vi "CAN_parse_BMS_1.vi"(11 "CAN message data":u8[](array[numeric])) -> ()   [LabVIEW 2018]
uses:
  Type_Def/TypeDef_BMSDatas.ctl
  Type_Def/TypeDef_BMSStatuss.ctl
  <vilib>/CANopenLib/CANOPEN.llb/CANopen Fetch from Data [U16].vi
  <vilib>/CANopenLib/CANOPEN.llb/CANopen Fetch from Data [I8].vi
panel:
  out "output cluster":T1
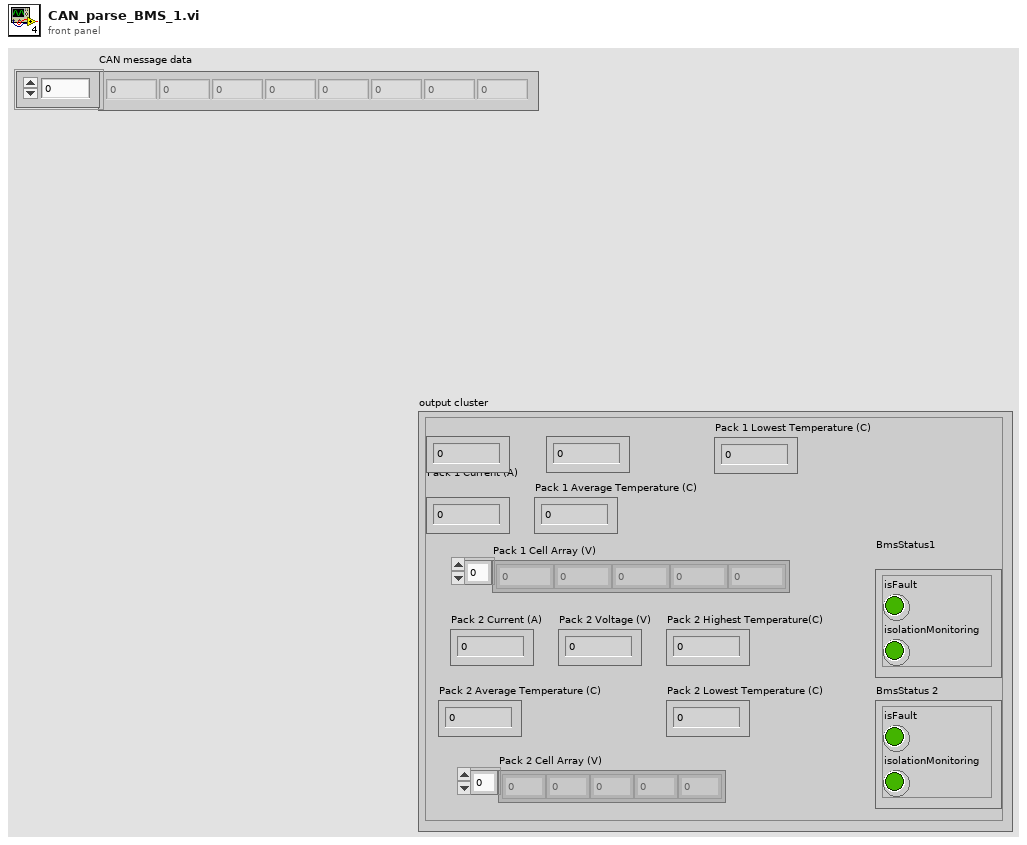
[diagram p1: front panel]
types:
  T1 = typedef "TypeDef_BMSDatas.ctl" = cluster{"Pack 1 Current (A)":dbl, "Pack 1 Voltage (V)":dbl, "Pack 1 Highest Temperature(C)":dbl, "BmsStatus1":T2, "Pack 2 Current (A)":dbl, "Pack 2 Voltage (V) ":dbl, "Pack 2 Highest Temperature(C) ":dbl, "BmsStatus 2":T2, "Pack 1 Cell Array (V)":dbl[], "Pack 2 Cell Array (V)":dbl[], "Pack 1 Lowest Temperature (C)":dbl, "Pack 1 Average Temperature (C)":dbl, "Pack 2 Average Temperature (C)":dbl, "Pack 2 Lowest Temperature (C)":dbl}
  T2 = typedef "TypeDef_BMSStatuss.ctl" = cluster{"isFault":bool, "isolationMonitoring":bool}
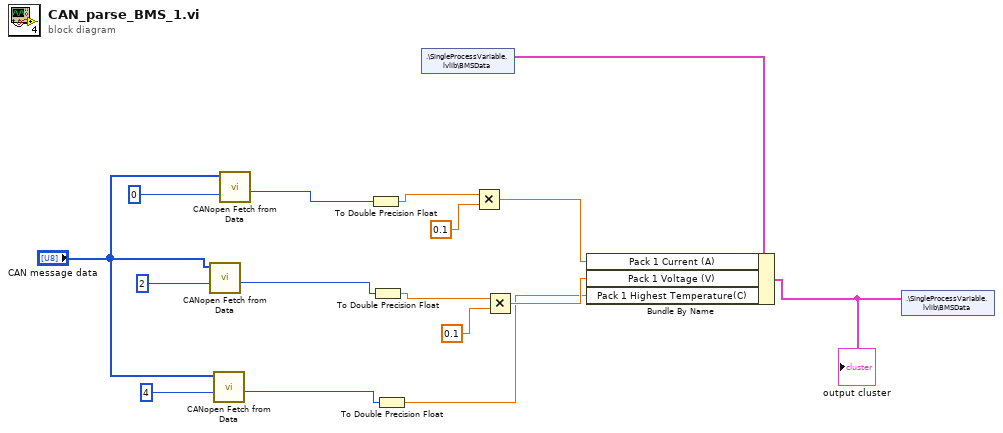
[diagram p0: block diagram]
diagram:
  n1 = call-poly <vilib>:"CANopen Fetch from Data.vi"("offset (0)"=2, "CANopen data in"="CAN message data") -> ("unsigned 16-bit integer"=w5:u16)  [unwired: 7 in, 2 out]
  n2 = call-poly <vilib>:"CANopen Fetch from Data.vi"("offset (0)"=4, "CANopen data in"="CAN message data") -> ("signed 8-bit integer"=w3:i8)  [unwired: 7 in, 2 out]
  n3 = call-poly <vilib>:"CANopen Fetch from Data.vi"("offset (0)"=0, "CANopen data in"="CAN message data") -> ("unsigned 16-bit integer"=w9:u16)  [unwired: 7 in, 2 out]
  n4 = To Double Precision Float(number=w9) -> (double precision float=w12:dbl)
  n5 = To Double Precision Float(number=w5) -> (double precision float=w6:dbl)
  n6 = To Double Precision Float(number=w3) -> (double precision float=w2:dbl)
  n7 = shared-variable ".\\SingleProcessVariable.lvlib\\BMSData"() -> (w14:T1)  [unwired: 1 in, 1 out]
  n8 = Multiply(x=w12, y=0.1) -> (x*y=w10:dbl)
  n9 = Multiply(x=w6, y=0.1) -> (x*y=w11:dbl)
  n10 = Bundle By Name(cluster=w14, "Pack 1 Current (A)"=w10, "Pack 1 Voltage (V)"=w11, "Pack 1 Highest Temperature(C)"=w2) -> (w13:T1)
  "output cluster" <- w13
  n11 = shared-variable ".\\SingleProcessVariable.lvlib\\BMSData"(w13) -> ()  [unwired: 1 in, 1 out]
